vi "Close.vi"(8 "error in (no error)":errorcluster, 11 "NhRegenGridSim in":refnum<class "NhRegenGridSim.lvclass">) -> (0 "error out":errorcluster, 3 "NhRegenGridSim out":refnum<class "NhRegenGridSim.lvclass">)   [LabVIEW 2014, in "AcPwrPlugins.lvlib" / "NhRegenGridSim.lvclass"]
uses:
  NhRegenGridSim.lvclass
  AcPwrBaseClass/AcPwrBase.lvclass/AcPwrBase.ctl
  AcPwrBaseClass/Accessors/Read Phases.vi
  <instrlib>/NH Research 9400 Series/NH Research 9400 Series.lvlib
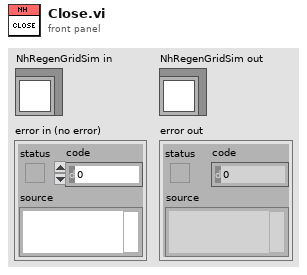
[diagram p1: front panel]
types:
  T1 = typedef "AcPwrPlugins.lvlib/AcPwrBase.lvclass/Phase.ctl" = cluster{"Enabled":bool, "VoltageLevel":dbl, "Waveform":string, "Name":string, "VoltageRange":dbl[], "CurrentLimit":dbl, "Handle":string, "Connected":bool}
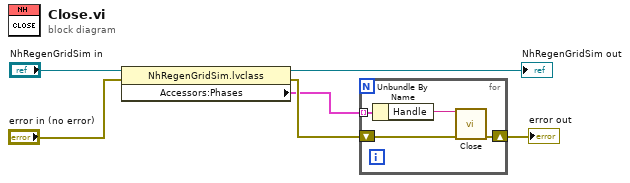
[diagram p0: block diagram]
diagram:
  n1 = property class="NhRegenGridSim.lvclass"(reference="NhRegenGridSim in", error in="error in (no error)") -> (reference out=→"NhRegenGridSim out":refnum<class "NhRegenGridSim.lvclass">, error out=w2:errorcluster, "Accessors:Phases"=w1:T1[])
  n2 = for {
    shift-right: [w10] -> w4
    shift-left: w2 -> [w9]
    tunnel: w1 -> [w8] mode=indexing
    n3 = Unbundle By Name(w8) -> ("Handle"=w7:string)
    n4 = call <instrlib>:"Close.vi"("VISA resource name"=w7, "error in (no error)"=w9) -> ("error out"=w10:errorcluster)  [unwired: 13 in]
  }
  "error out" <- w4
